vi "girpcutil_ClearValues.vi"(8 "Fehler (Eingang, kein Fehler)":errorcluster, 11 "girpcutil_params":T1) -> (0 "error IO":errorcluster)   [LabVIEW 2016]
uses:
  girpcutil_params.ctl
panel:
  out "errMsg":u8[](array[numeric])
  out "errMsgLen":i32
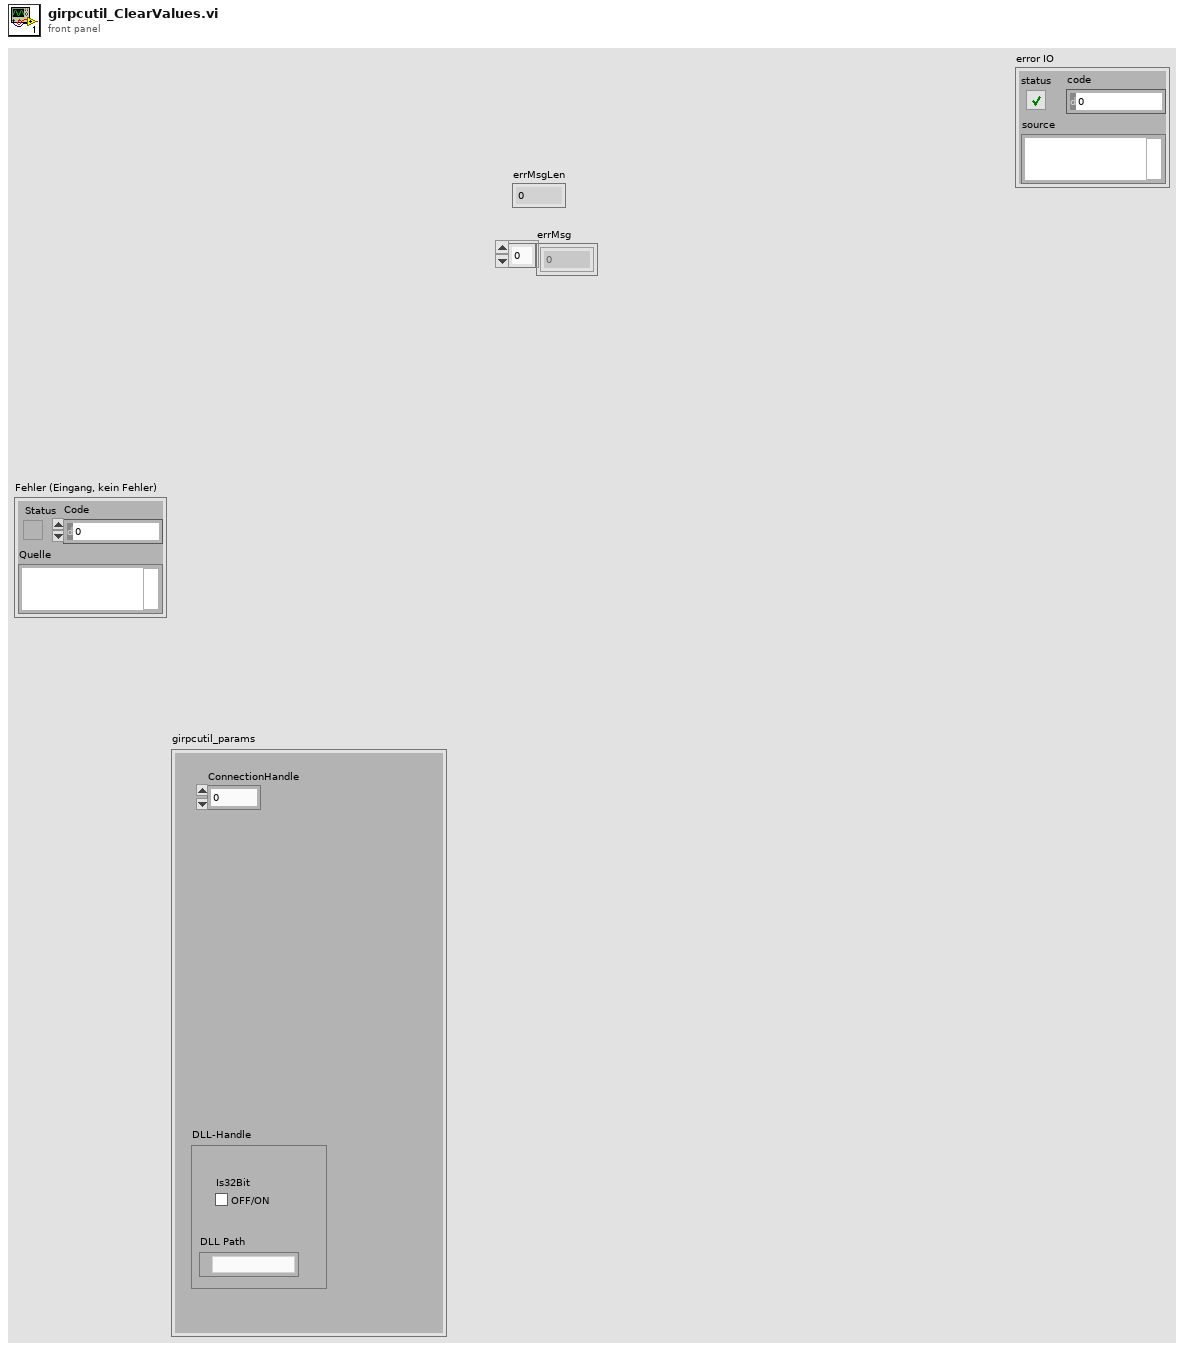
[diagram p1: front panel]
types:
  T1 = typedef "girpcutil_params.ctl" = cluster{"ConnectionHandle":i32, "DLL-Handle":cluster{"DLL Path":path, "Is32Bit":bool}}
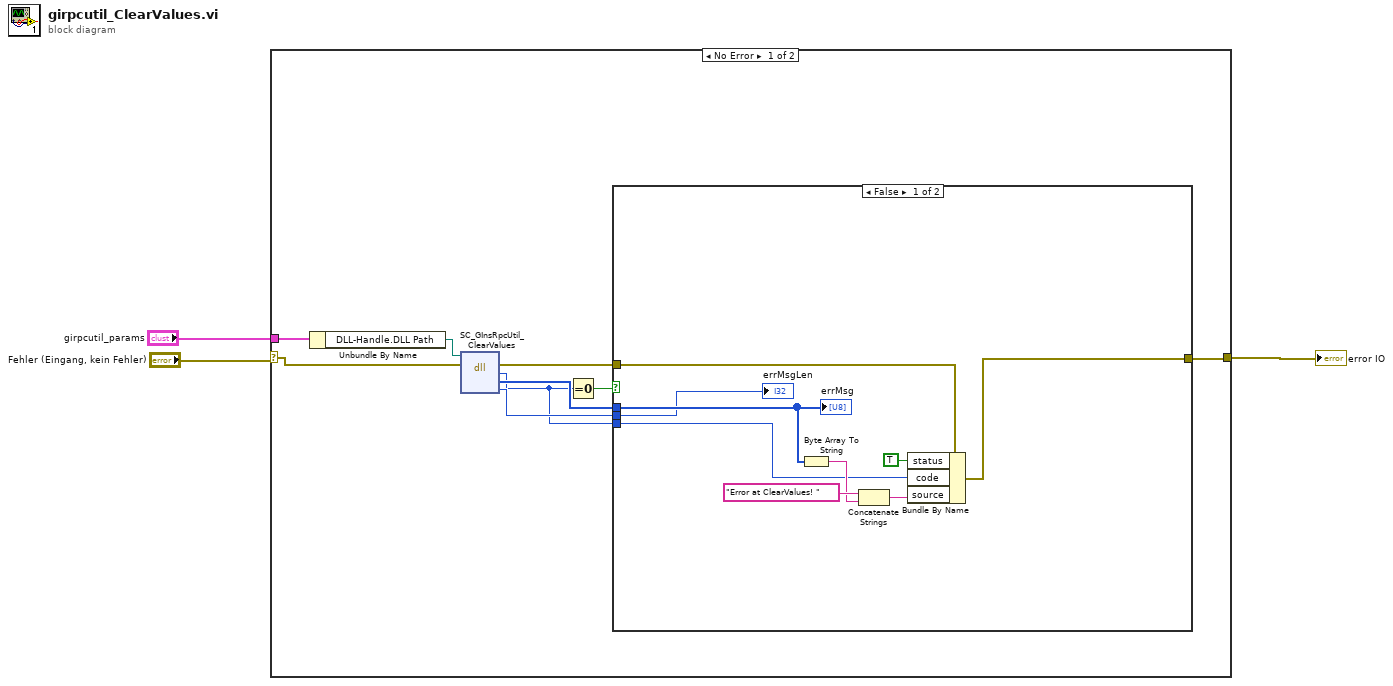
[diagram p0: block diagram]
diagram:
  n1 = case shown="No Error" "Fehler (Eingang, kein Fehler)" {
    selector: "Fehler (Eingang, kein Fehler)" -> [w11 w23]
    tunnel: [w4 w23] -> w2
    tunnel: "girpcutil_params" -> [w12 _]
    frame No Error {
      n2 = Unbundle By Name(w12) -> ("DLL-Handle.DLL Path"=w10:path)
      n3 = dll-call lib="?" fn="SC_GInsRpcUtil_ClearValues"(path in=w10, error in=w11) -> (error out=w9:errorcluster, "Rückgabewert"=w5:i32, "errMsg"=w7:u8[], "errMsgLen"=w6:i32)  [unwired: 3 in, 1 out]
      n4 = Equal To 0?(x=w5) -> (x = 0?=w8:bool)
      n5 = case shown="False" w8 {
        tunnel: [w15 w22] -> w4
        tunnel: w7 -> [w19 _]
        tunnel: w6 -> [w16 _]
        tunnel: w5 -> [w14 _]
        tunnel: w9 -> [w13 w22]
        frame False {
          n6 = Byte Array To String(unsigned byte array=w19) -> (string=w20:string)
          n7 = Concatenate Strings("Error at ClearValues! " ("source"), w20) -> (w18:string)
          n8 = Bundle By Name(cluster=w13, "status"=TRUE, "code"=w14, "source"=w18) -> (w15:errorcluster)
          "errMsg" <- w19
          "errMsgLen" <- w16
        }
        frame True {
        }
      }
    }
    frame Error {
    }
  }
  "error IO" <- w2
